vi "Set Node Text Content.vi"(8 "error in (no error)":errorcluster, 10 "node text":string, 11 "node in":refnum<k20>) -> (0 "error out":errorcluster, 3 "node out":refnum<k20>)   [LabVIEW 2017, in "Error File Management.lvlib"]
uses:
  Error File Management.lvlib
  <vilib>/xml/Close Reference(Node).vi
  <resource>/objmgr/DOMUserDefRef.rc
  <vilib>/xml/NI_XML.lvlib
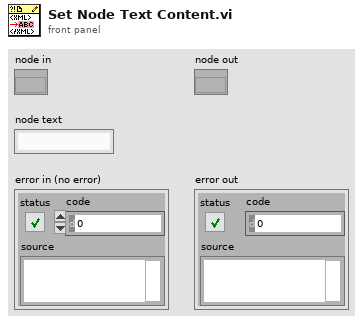
[diagram p1: front panel]
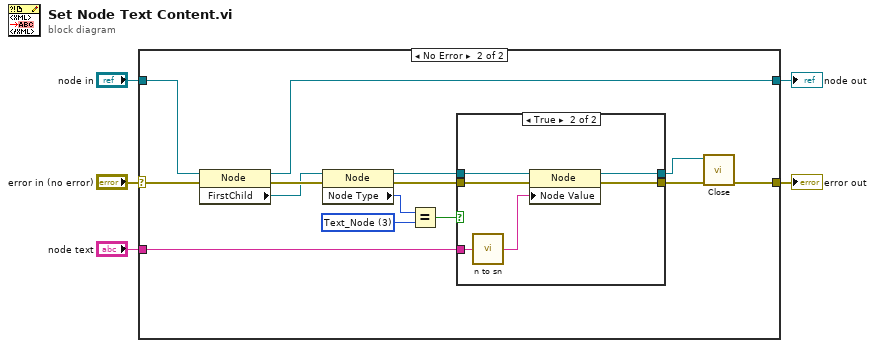
[diagram p0: block diagram]
diagram:
  n1 = case shown="No Error" "error in (no error)" {
    selector: "error in (no error)" -> [w7 w16]
    tunnel: "node in" -> [w6 w21]
    tunnel: [w6 w18] -> w4
    tunnel: "node text" -> [_ w15]
    tunnel: [w7 w17] -> w1
    frame Error {
    }
    frame No Error {
      w13 = 3 items=["Element_Node"=1, "Attribute_Node"=2, "Text_Node"=3, "CDATASection_Node"=4, "EntityReference_Node"=5, "Entity_Node"=6, "ProcessingInstruction_Node"=7, "Comment_Node"=8, "Document_Node"=9, "DocumentType_Node"=10, "DocumentFragment_Node"=11, "Notation_Node"=12] ("Node Type")
      n2 = property on="Property Node" class="Node"(reference=w21, error in=w16) -> (reference out=w18:refnum<k20>, error out=w20:errorcluster, "FirstChild"=w19:refnum<k20>)
      n3 = property class="Node"(reference=w19, error in=w20) -> (reference out=w11:refnum<k20>, error out=w10:errorcluster, "Node Type"=w14:i32)
      n4 = Equal?(x=w14, y=w13) -> (x = y?=w12:bool)
      n5 = case shown="True" w12 {
        tunnel: w11 -> [w23 w29]
        tunnel: w10 -> [w22 w28]
        tunnel: [w23 w27] -> w9
        tunnel: [w22 w26] -> w8
        tunnel: w15 -> [_ w25]
        frame False {
        }
        frame True {
          n6 = call "n to sn.vi"("in"=w25) -> ("out"=w24:string)
          n7 = property class="Node"(reference=w29, error in=w28, "Node Value"=w24) -> (reference out=w27:refnum<k20>, error out=w26:errorcluster)
        }
      }
      n8 = call-poly <vilib>:"Close.vi"("error in (no error)"=w8, "node"=w9) -> ("error out"=w17:errorcluster)  [unwired: 7 out]
    }
  }
  "node out" <- w4
  "error out" <- w1
